vi "capex scheduler.vi"(11 "Path":path=path "C:/NI projects/Chamber control labview") -> ()   [LabVIEW 2013]
uses:
  <instrlib>/APS-7000 Series/APS-7000 Series.lvlib
panel:
  in  "DC PS timeout":i32
  in  "AC PS timeout":i32
  in  "Relays":i32=10
  in  "Analog in":i32=10
  in  "GPIO":i32=10
  # "All times in milliseconds between executions"
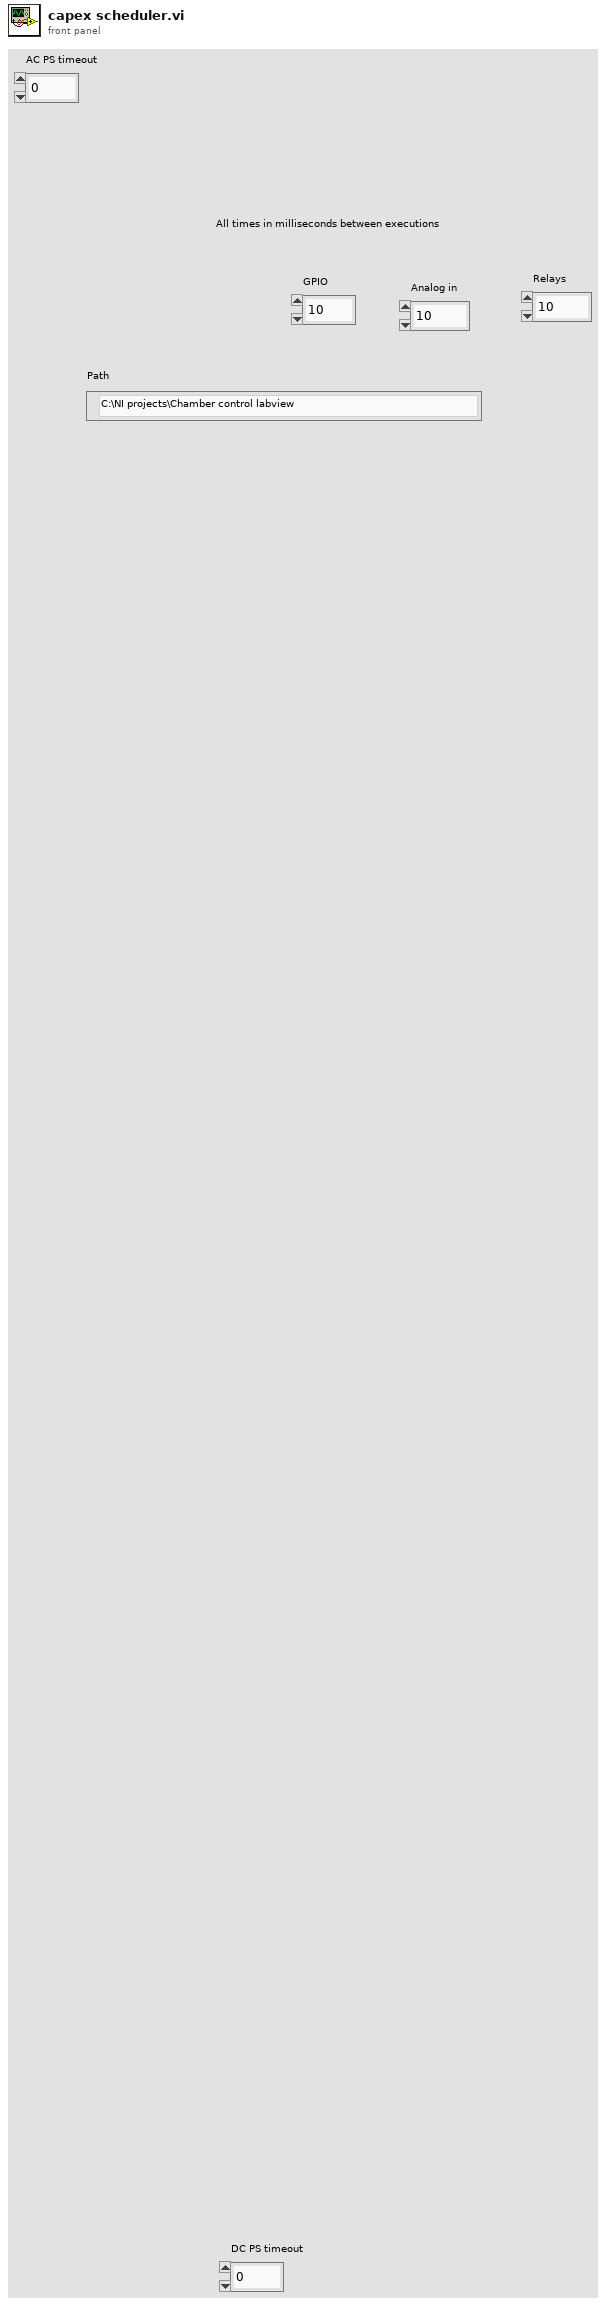
[diagram p1: front panel]
types:
  T1 = enum16{"Chiller", "Chamber", "DC power", "AC power", "GPIO", "temperature", "relays", "analog"}
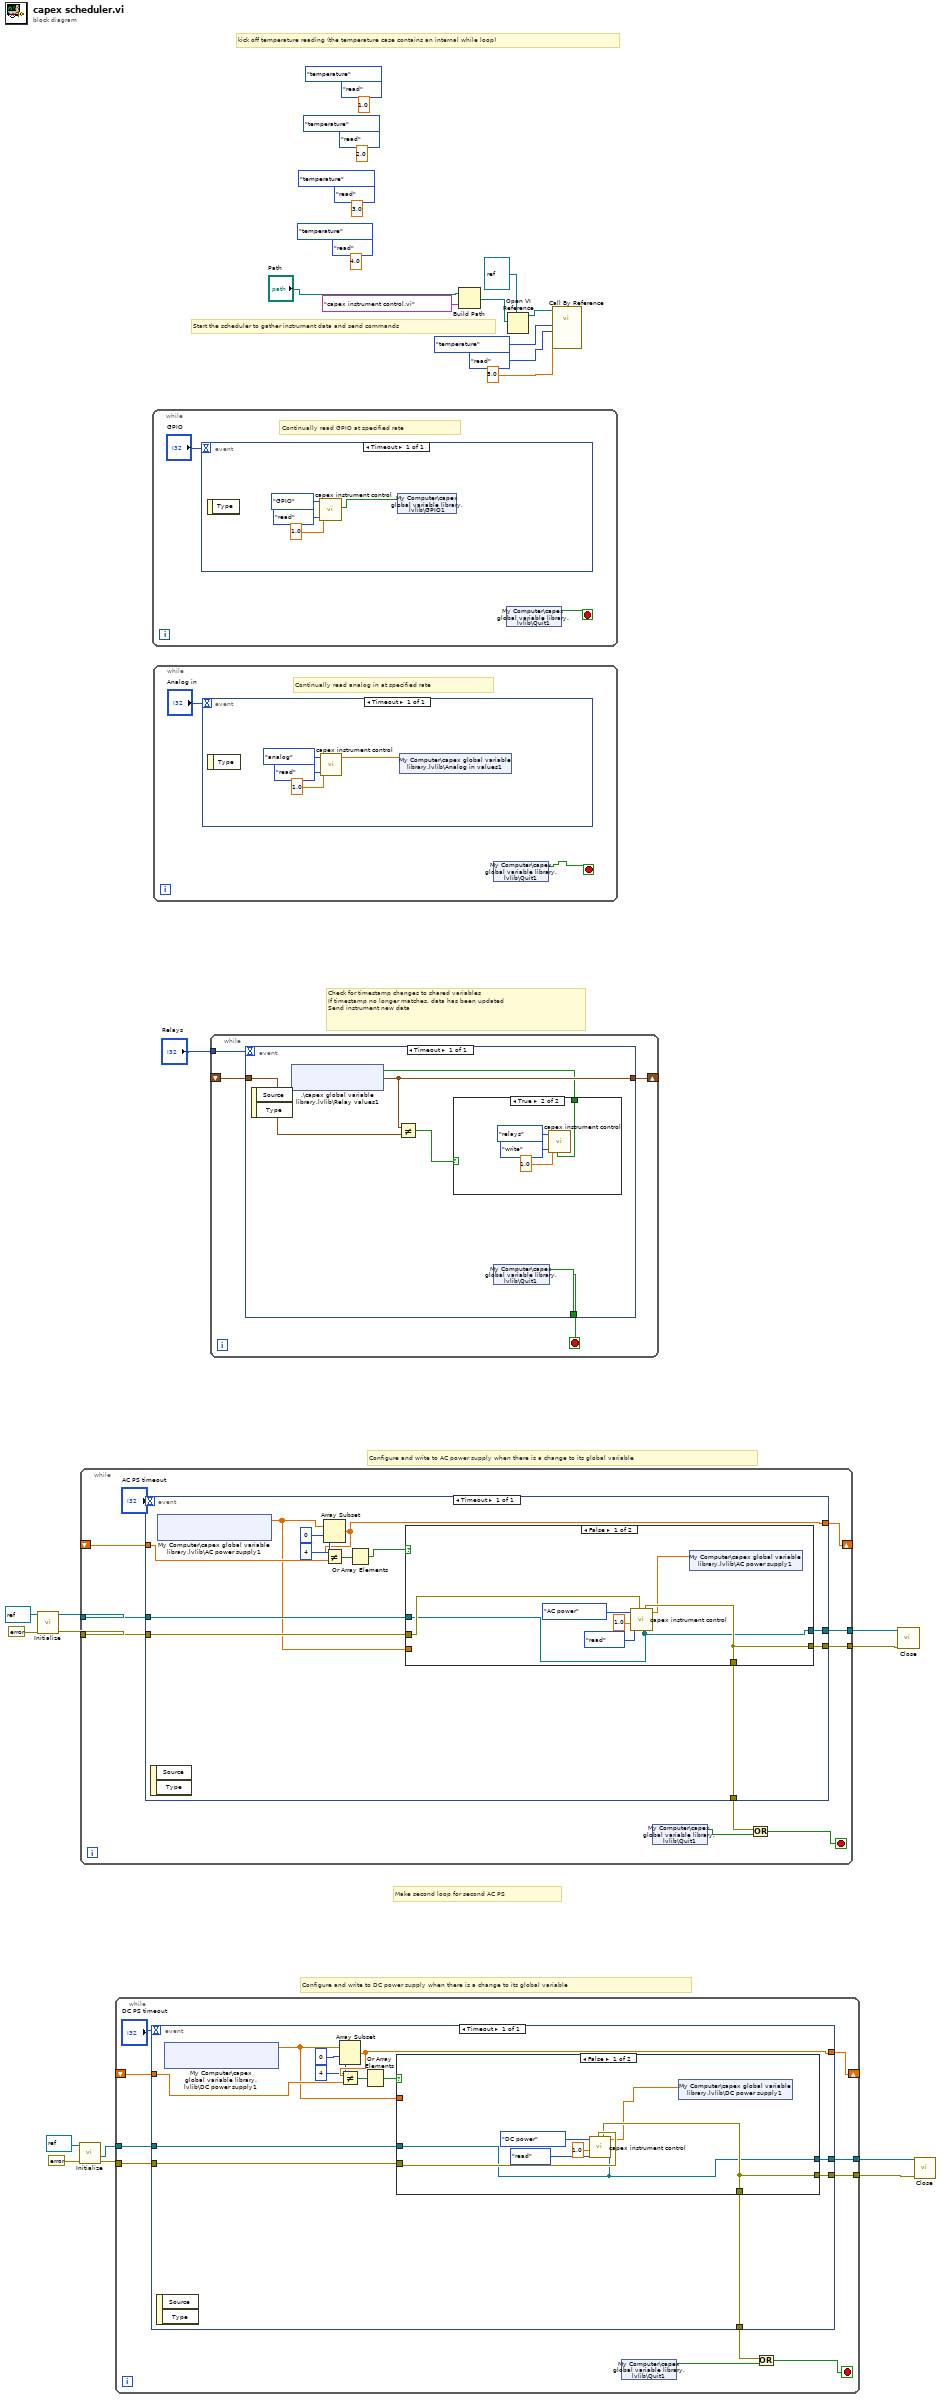
[diagram p0: block diagram]
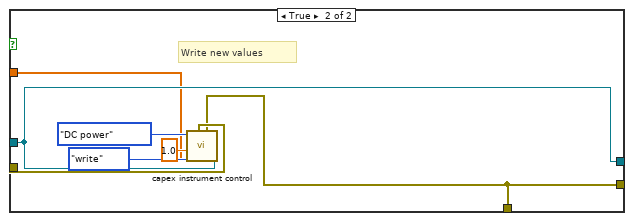
[diagram p2: hidden frame]
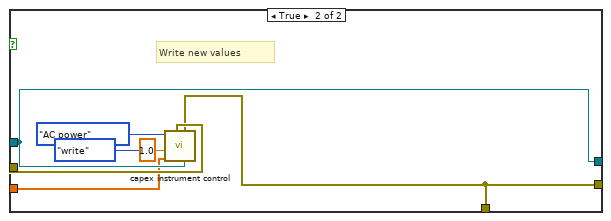
[diagram p3: hidden frame]
diagram:
  (unwired) 4.0 ("Module")
  (unwired) enum16{"read", "write"}."read" ("read/write")
  (unwired) T1."temperature" ("Subsystem")
  (unwired) 3.0 ("Module")
  (unwired) enum16{"read", "write"}."read" ("read/write")
  (unwired) T1."temperature" ("Subsystem")
  (unwired) 2.0 ("Module")
  (unwired) enum16{"read", "write"}."read" ("read/write")
  (unwired) T1."temperature" ("Subsystem")
  (unwired) 1.0 ("Module")
  (unwired) enum16{"read", "write"}."read" ("read/write")
  (unwired) T1."temperature" ("Subsystem")
  # "Configure and write to DC power supply when there is a change to its global variable"
  # "Make second loop for second AC PS"
  # "Configure and write to AC power supply when there is a change to its global variable"
  # "Start the scheduler to gather instrument data and send commands"
  # "kick off temperature reading (the temperature case contains an internal while loop)"
  # "Check for timestamp changes to shared variables\nIf timestamp no longer matches, data has been updated\nSend instrument new data"
  n1 = call <instrlib>:"Initialize.vi"("error in (no error)"=errorcluster {"status"=FALSE, "code"=0, "source"=""}, "VISA resource name"=refnum<visa-resource-name> refnum) -> ("error out"=w8:errorcluster, "VISA resource name out"=w11:refnum<visa-resource-name>)  [unwired: 8 in]
  n2 = call <instrlib>:"Initialize.vi"("error in"=errorcluster {"status"=FALSE, "code"=0, "source"=""} ("error in (no error)"), "VISAIn"=refnum<visa-resource-name> refnum ("VISA resource name")) -> ("ErrorOut"=w3:errorcluster, "Keithley2268Lib.IKeithley2268"=w2:refnum<k7>)  [unwired: 7 in, 1 out]
  n3 = while {
    shift-right: [w30] -> _
    shift-left: _ -> [w31]
    tunnel: w11 -> [w27]
    tunnel: [w26] -> w10
    tunnel: w8 -> [w25]
    tunnel: [w24] -> w7
    stop <- w29 stop-if-true
    n4 = event shown="[0] Timeout" {
      selector: _ -> [_]
      dyn-events: _ -> [_]
      timeout: "AC PS timeout" -> [_]
      tunnel: w31 -> [w34]
      tunnel: [w35] -> w30
      tunnel: [w43] -> w28
      tunnel: w27 -> [w42]
      tunnel: [w41] -> w26
      tunnel: w25 -> [w40]
      tunnel: [w39] -> w24
      event Timeout {
        n5 = event-data() -> ()  [unwired: 1 in, 2 out]
        n6 = shared-variable "My Computer\\capex global variable library.lvlib\\AC power supply1"() -> (w32:dbl[])  [unwired: 1 in, 2 out]
        n7 = Array Subset(array=w32, index=0, length=4) -> (w35:dbl[])
        n8 = Not Equal?(x=w35, y=w34) -> (x != y?=w36:bool[])
        n9 = Or Array Elements(Boolean array=w36) -> (logical OR=w33:bool)
        n10 = case shown="False" w33 {
          tunnel: [w47 w56] -> w43
          tunnel: w42 -> [w45 w55]
          tunnel: [w45 w55] -> w41
          tunnel: w40 -> [w46 w57]
          tunnel: [w47 w56] -> w39
          tunnel: w32 -> [_ w51]
          frame False {
            n11 = call "capex instrument control.vi"("VISA resource name"=w45, "error in"=w46, "Module"=1.0, "read/write"=enum16{"read", "write"}."read", "Subsystem"=T1."AC power") -> ("Value out"=w44:dbl[], "error out"=w47:errorcluster)  [unwired: 4 in, 1 out]
            n12 = shared-variable "My Computer\\capex global variable library.lvlib\\AC power supply1"(w44) -> ()  [unwired: 1 in, 1 out]
          }
          frame True {
            # "Write new values"
            n13 = call "capex instrument control.vi"("VISA resource name"=w55, "error in"=w57, "Value in"=w51, "Module"=1.0, "read/write"=enum16{"read", "write"}."write", "Subsystem"=T1."AC power") -> ("error out"=w56:errorcluster)  [unwired: 3 in, 2 out]
          }
        }
      }
    }
    n14 = shared-variable "My Computer\\capex global variable library.lvlib\\Quit1"() -> (w22:bool)  [unwired: 1 in, 1 out]
    n15 = Or(x=w28, y=w22) -> (x .or. y?=w29:bool)
  }
  n16 = while {
    shift-right: [w66] -> _
    shift-left: _ -> [w67]
    tunnel: w2 -> [w63]
    tunnel: [w62] -> w1
    tunnel: w3 -> [w61]
    tunnel: [w60] -> w6
    stop <- w65 stop-if-true
    n17 = event shown="[0] Timeout" {
      selector: _ -> [_]
      dyn-events: _ -> [_]
      timeout: "DC PS timeout" -> [_]
      tunnel: w67 -> [w79]
      tunnel: [w73] -> w66
      tunnel: [w78] -> w64
      tunnel: w63 -> [w77]
      tunnel: [w76] -> w62
      tunnel: w61 -> [w75]
      tunnel: [w74] -> w60
      event Timeout {
        n18 = event-data() -> ()  [unwired: 1 in, 2 out]
        n19 = shared-variable "My Computer\\capex global variable library.lvlib\\DC power supply1"() -> (w68:dbl[])  [unwired: 1 in, 2 out]
        n20 = Array Subset(array=w68, index=0, length=4) -> (w73:dbl[])
        n21 = Not Equal?(x=w73, y=w79) -> (x != y?=w70:bool[])
        n22 = Or Array Elements(Boolean array=w70) -> (logical OR=w69:bool)
        n23 = case shown="False" w69 {
          tunnel: [w82 w92] -> w78
          tunnel: w77 -> [w80 w89]
          tunnel: [w80 w89] -> w76
          tunnel: w75 -> [w83 w93]
          tunnel: [w82 w92] -> w74
          tunnel: w68 -> [_ w87]
          frame False {
            n24 = call "capex instrument control.vi"("Keithley2268Lib.IKeithley2268"=w80, "error in"=w83, "Module"=1.0, "read/write"=enum16{"read", "write"}."read", "Subsystem"=T1."DC power") -> ("Value out"=w81:dbl[], "error out"=w82:errorcluster)  [unwired: 4 in, 1 out]
            n25 = shared-variable "My Computer\\capex global variable library.lvlib\\DC power supply1"(w81) -> ()  [unwired: 1 in, 1 out]
          }
          frame True {
            # "Write new values"
            n26 = call "capex instrument control.vi"("Keithley2268Lib.IKeithley2268"=w89, "error in"=w93, "Value in"=w87, "Module"=1.0, "read/write"=enum16{"read", "write"}."write", "Subsystem"=T1."DC power") -> ("error out"=w92:errorcluster)  [unwired: 3 in, 2 out]
          }
        }
      }
    }
    n27 = shared-variable "My Computer\\capex global variable library.lvlib\\Quit1"() -> (w58:bool)  [unwired: 1 in, 1 out]
    n28 = Or(x=w64, y=w58) -> (x .or. y?=w65:bool)
  }
  n29 = while {
    stop <- w94 stop-if-true
    # "Continually read GPIO at specified rate"
    n30 = event shown="[0] Timeout" {
      selector: _ -> [_]
      dyn-events: _ -> [_]
      timeout: "GPIO" -> [_]
      event Timeout {
        n31 = event-data() -> ()  [unwired: 1 in, 1 out]
        n32 = call "capex instrument control.vi"("Module"=1.0, "read/write"=enum16{"read", "write"}."read", "Subsystem"=T1."GPIO") -> ("Bool out"=w96:bool[])  [unwired: 6 in, 2 out]
        n33 = shared-variable "My Computer\\capex global variable library.lvlib\\GPIO1"(w96) -> ()  [unwired: 1 in, 1 out]
      }
    }
    n34 = shared-variable "My Computer\\capex global variable library.lvlib\\Quit1"() -> (w94:bool)  [unwired: 1 in, 1 out]
  }
  n35 = while {
    stop <- w100 stop-if-true
    # "Continually read analog in at specified rate"
    n36 = event shown="[0] Timeout" {
      selector: _ -> [_]
      dyn-events: _ -> [_]
      timeout: "Analog in" -> [_]
      event Timeout {
        n37 = event-data() -> ()  [unwired: 1 in, 1 out]
        n38 = call "capex instrument control.vi"("Module"=1.0, "read/write"=enum16{"read", "write"}."read", "Subsystem"=T1."analog") -> ("Value out"=w102:dbl[])  [unwired: 6 in, 2 out]
        n39 = shared-variable "My Computer\\capex global variable library.lvlib\\Analog in values1"(w102) -> ()  [unwired: 1 in, 1 out]
      }
    }
    n40 = shared-variable "My Computer\\capex global variable library.lvlib\\Quit1"() -> (w100:bool)  [unwired: 1 in, 1 out]
  }
  n41 = while {
    shift-right: [w108] -> _
    shift-left: _ -> [w109]
    tunnel: "Relays" -> [w106]
    stop <- w107 stop-if-true
    n42 = event shown="[0] Timeout" {
      selector: _ -> [_]
      dyn-events: _ -> [_]
      timeout: w106 -> [_]
      tunnel: w109 -> [w114]
      tunnel: [w113] -> w108
      tunnel: [w110] -> w107
      event Timeout {
        n43 = event-data() -> ()  [unwired: 1 in, 2 out]
        n44 = shared-variable ".\\capex global variable library.lvlib\\Relay values1"() -> (w111:bool[], w113:timestamp)  [unwired: 1 in, 1 out]
        n45 = Not Equal?(x=w113, y=w114) -> (x != y?=w112:bool)
        n46 = case shown="True" w112 {
          tunnel: w111 -> [_ w115]
          frame False {
          }
          frame True {
            n47 = call "capex instrument control.vi"("Bool in"=w115, "Module"=1.0, "read/write"=enum16{"read", "write"}."write", "Subsystem"=T1."relays") -> ()  [unwired: 5 in, 3 out]
          }
        }
        n48 = shared-variable "My Computer\\capex global variable library.lvlib\\Quit1"() -> (w110:bool)  [unwired: 1 in, 1 out]
      }
    }
  }
  n49 = Build Path(base path="Path", name or relative path="capex instrument control.vi") -> (appended path=w14:path)
  n50 = Open VI Reference(type specifier VI Refnum (for type only)=refnum<vi> refnum, vi path=w14) -> (vi reference=w16:refnum<vi>)  [unwired: 4 in, 1 out]
  n51 = call-by-ref "?"(reference=w16, "Module"=5.0, "read/write"=enum16{"read", "write"}."read", "Subsystem"=T1."temperature") -> ()  [unwired: 8 in, 4 out]
  n52 = call <instrlib>:"Close.vi"("error in (no error)"=w7, "VISA resource name"=w10) -> ()  [unwired: 9 in, 1 out]
  n53 = call <instrlib>:"Close.vi"("error in (no error)"=w6, "Keithley2268Lib.IKeithley2268"=w1) -> ()  [unwired: 9 in, 1 out]
